vi "Find & Connect Terminals.vi"(7 "Id":string, 8 "error in (no error)":errorcluster, 9 "Terms":T1, 10 "Terms IDs":T4[](array[typedef]), 11 "Wire Source":refnum<vi>) -> (0 "error out":errorcluster)   [LabVIEW 2016, in "LV Object Event Registration Node.xnode"]
uses:
  LV Object Event Registration Node.xnode
  <vilib>/XNodeSupport/XNodeString.ctl
  <vilib>/XNodeSupport/XNodeTermIDPairs.ctl
  <vilib>/XNodeSupport/XNodeTermIDPair.ctl
  <vilib>/XNodeSupport/XNodeTermRef.ctl
  <vilib>/XNodeSupport/NI_XNodeSupport.lvlib
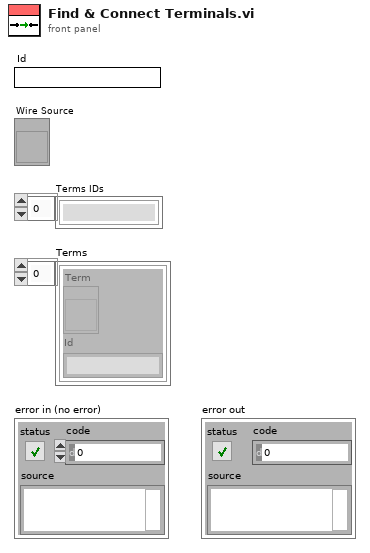
[diagram p1: front panel]
types:
  T1 = typedef "NI_XNodeSupport.lvlib/XNodeTermIDPairs.ctl" = T2[]
  T2 = typedef "NI_XNodeSupport.lvlib/XNodeTermIDPair.ctl" = cluster{"Term":T3, "Id":T4}
  T3 = typedef "NI_XNodeSupport.lvlib/XNodeTermRef.ctl" = refnum<vi>
  T4 = typedef "NI_XNodeSupport.lvlib/XNodeString.ctl" = string
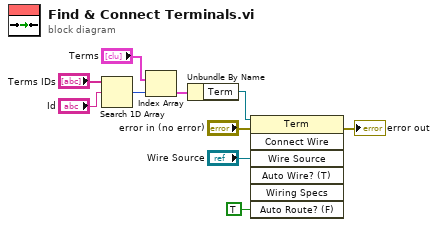
[diagram p0: block diagram]
diagram:
  n1 = Search 1D Array(1D array="Terms IDs", element="Id") -> (index of element=w3:i32)  [unwired: 1 in]
  n2 = Index Array(array="Terms", index=w3) -> (element=w4:T2)
  n3 = Unbundle By Name(w4) -> ("Term"=w5:T3)
  n4 = invoke class="Term" method="Connect Wire"(reference=w5, error in="error in (no error)", "Wire Source"="Wire Source", "Auto Route? (F)"=TRUE) -> (error out=→"error out":errorcluster)  [unwired: 3 in, 6 out]
